vi "find_patches.vi"(5 "Shrink Factor":i32=1, 6 "Field of View":cluster{"fieldOfViewX":sgl, "fieldOfViewY":sgl}, 8 "error in":errorcluster, 10 "find_patches parameters":T2, 11 "Image":T3) -> (0 "error out":errorcluster, 2 "Patches":T1(array[cluster]))   [LabVIEW 2024, in "Vision.lvlib"]
uses:
  Vision.lvlib
  <vilib>/vision/Image Controls.llb/IMAQ Image.ctl
  find_patches parameters.ctl
  bin/PatternRecognition.dll
panel:
  # "Image must be an 8-bin greyscale image"
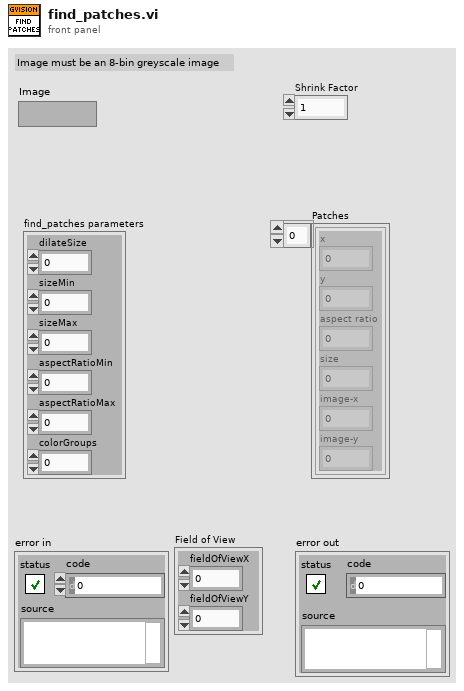
[diagram p1: front panel]
types:
  T1 = cluster{"x":dbl, "y":dbl, "aspect ratio":dbl, "size":dbl, "image-x":dbl, "image-y":dbl}[]
  T2 = typedef "Vision.lvlib/find_patches parameters.ctl" = cluster{"dilateSize":i32, "sizeMin":sgl, "sizeMax":sgl, "aspectRatioMin":sgl, "aspectRatioMax":sgl, "colorGroups":i32}
  T3 = typedef "IMAQ Image.ctl" = refnum<image>
  T4 = enum32{"Map Pixel Pointer", "Unmap Pixel Pointer", "Get Pixels Infos"}
  T5 = cluster{"x":dbl, "y":dbl, "aspect ratio":dbl, "size":dbl, "image-x":dbl, "image-y":dbl}
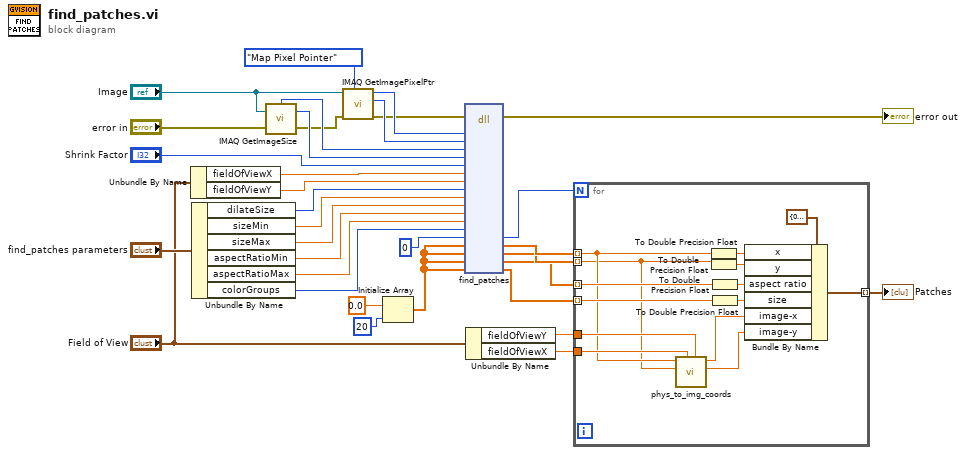
[diagram p0: block diagram]
diagram:
  n1 = Unbundle By Name("Field of View") -> ("fieldOfViewX"=w2:sgl, "fieldOfViewY"=w1:sgl)
  n2 = Unbundle By Name("find_patches parameters") -> ("dilateSize"=w25:i32, "sizeMin"=w24:sgl, "sizeMax"=w23:sgl, "aspectRatioMin"=w22:sgl, "aspectRatioMax"=w21:sgl, "colorGroups"=w20:i32)
  n3 = call "IMAQ GetImageSize"("Image"="Image", "error in (no error)"="error in") -> ("Y Resolution"=w9:i32, "X Resolution"=w10:i32, "error out"=w8:errorcluster)  [unwired: 2 in]
  n4 = call "IMAQ GetImagePixelPtr"("Function"=T4."Map Pixel Pointer", "error in (no error)"=w8, "Image"="Image") -> ("error out"=w14:errorcluster, "LineWidth(Pixels)"=w27:i32, "Pixel Pointer out"=w28:u64)  [unwired: 3 in, 3 out]
  n5 = Initialize Array(sgl 0.0 ("element"), 20 ("dimension size")) -> (w19:sgl[])
  n6 = dll-call lib="C:/Users/cfang/Desktop/nebraska-silicon-lab/pixel-gantry-control/Gantry/Shared Components/bin/PatternRecognition.dll" fn="find_patches"(error in=w14, "imgPtr"=w28, "imgLineWidth"=w27, "imgWidth"=w10, "imgHeight"=w9, "shrinkFactor"="Shrink Factor", "fieldOfViewX"=w2, "fieldOfViewY"=w1, "dilateSize"=w25, "sizeMin"=w24, "sizeMax"=w23, "aspectRatioMin"=w22, "aspectRatioMax"=w21, "colorGroups"=w20, "numPatches"=0 ("numFiducials"), "patchXCoordinates"=w19, "patchYCoordinates"=w19, "patchAspectRatios"=w19, "patchSizes"=w19) -> (error out=→"error out":errorcluster, "numPatches"=w26:i32, "patchXCoordinates"=w18:sgl[], "patchYCoordinates"=w17:sgl[], "patchAspectRatios"=w16:sgl[], "patchSizes"=w15:sgl[])  [unwired: 16 in, 1 out]
  n7 = Unbundle By Name("Field of View") -> ("fieldOfViewY"=w6:sgl, "fieldOfViewX"=w5:sgl)
  n8 = for {
    N: w26 -> [_]
    tunnel: w18 -> [w37] mode=indexing
    tunnel: w17 -> [w36] mode=indexing
    tunnel: [w47] -> w4 mode=indexing
    tunnel: w16 -> [w42] mode=indexing
    tunnel: w15 -> [w41] mode=indexing
    tunnel: w6 -> [w39]
    tunnel: w5 -> [w38]
    n9 = call "phys_to_img_coords.vi"("fov_y"=w39, "fov_x"=w38, "y"=w36, "x"=w37) -> ("image_y"=w34:dbl, "image_x"=w35:dbl)  [unwired: 6 in]
    n10 = To Double Precision Float(number=w37) -> (double precision float=w46:dbl)
    n11 = To Double Precision Float(number=w36) -> (double precision float=w45:dbl)
    n12 = To Double Precision Float(number=w42) -> (double precision float=w44:dbl)
    n13 = To Double Precision Float(number=w41) -> (double precision float=w43:dbl)
    n14 = Bundle By Name(cluster=T5 {"x"=0.0, "y"=0.0, "aspect ratio"=0.0, "size"=0.0, "image-x"=0.0, "image-y"=0.0}, "x"=w46, "y"=w45, "aspect ratio"=w44, "size"=w43, "image-x"=w35, "image-y"=w34) -> (w47:T5)
  }
  "Patches" <- w4
